vi "Mode to ROI conversion.vi"(10 "Mode":dbl, 11 "Color":string) -> (3 "CCD ROI":cluster{i32, i32, i32, i32, i32, i32}={0, 4096, 1, 0, 4096, 1})   [LabVIEW 2015]
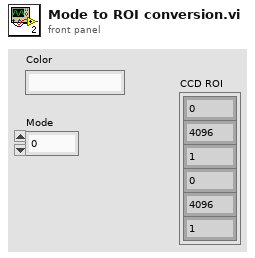
[diagram p1: front panel]
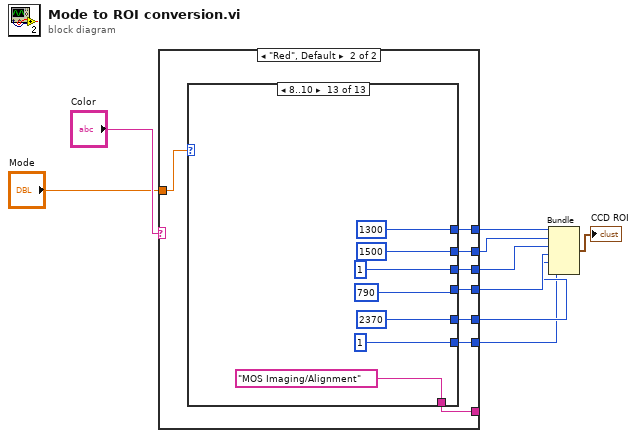
[diagram p0: block diagram]
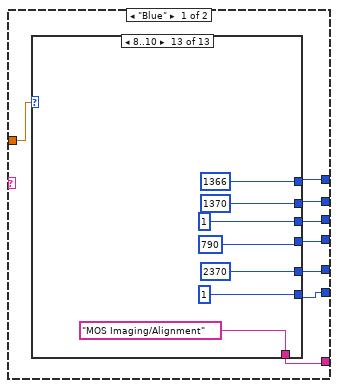
[diagram p2: hidden frame]
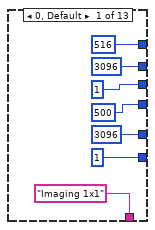
[diagram p3: hidden frame]
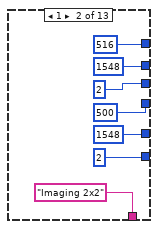
[diagram p4: hidden frame]
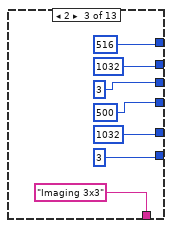
[diagram p5: hidden frame]
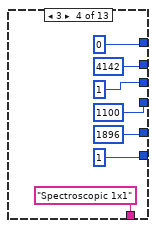
[diagram p6: hidden frame]
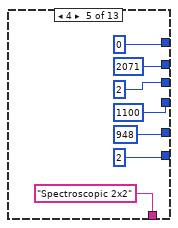
[diagram p7: hidden frame]
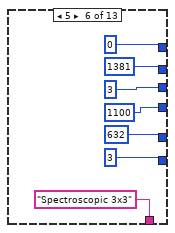
[diagram p8: hidden frame]
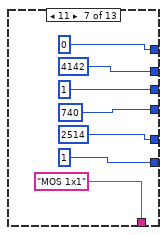
[diagram p9: hidden frame]
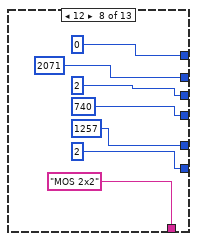
[diagram p10: hidden frame]
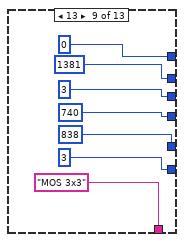
[diagram p11: hidden frame]
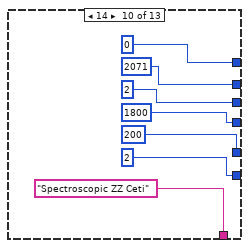
[diagram p12: hidden frame]
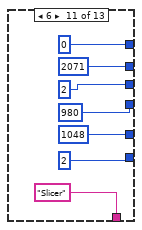
[diagram p13: hidden frame]
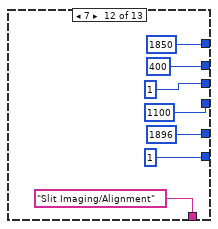
[diagram p14: hidden frame]
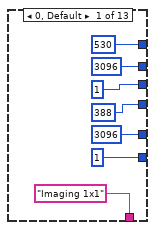
[diagram p15: hidden frame]
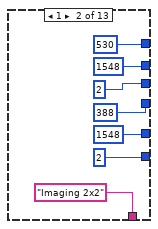
[diagram p16: hidden frame]
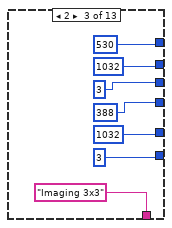
[diagram p17: hidden frame]
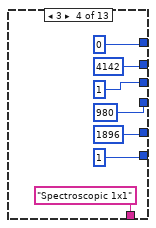
[diagram p18: hidden frame]
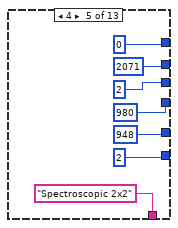
[diagram p19: hidden frame]
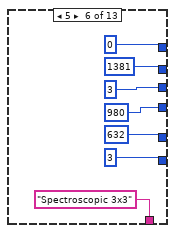
[diagram p20: hidden frame]
diagram:
  n1 = case shown="\"Red\", Default" "Color" {
    tunnel: [w14 w116] -> w6
    tunnel: [w13 w115] -> w5
    tunnel: [w12 w114] -> w4
    tunnel: [w11 w113] -> w3
    tunnel: [w15 w112] -> w2
    tunnel: [w16 w111] -> w1
    tunnel: [w17 w110] -> _
    tunnel: "Mode" -> [w10 w109]
    frame "Blue" {
      n2 = case shown="8..10" w10 {
        tunnel: [516 516 516 0 0 0 0 0 0 0 0 1850 1366] -> w14
        tunnel: [3096 1548 1032 4142 2071 1381 4142 2071 1381 2071 2071 400 1370] -> w13
        tunnel: [1 2 3 1 2 3 1 2 3 2 2 1 1] -> w12
        tunnel: [500 500 500 1100 1100 1100 740 740 740 1800 980 1100 790] -> w11
        tunnel: [3096 1548 1032 1896 948 632 2514 1257 838 200 1048 1896 2370] -> w15
        tunnel: [1 2 3 1 2 3 1 2 3 2 2 1 1] -> w16
        tunnel: ["Imaging 1x1" ("Current Status") "Imaging 2x2" ("Current Status") "Imaging 3x3" ("Current Status") "Spectroscopic 1x1" ("Current Status") "Spectroscopic 2x2" ("Current Status") "Spectroscopic 3x3" ("Current Status") "MOS 1x1" ("Current Status") "MOS 2x2" ("Current Status") "MOS 3x3" ("Current Status") "Spectroscopic ZZ Ceti" ("Current Status") "Slicer" ("Current Status") "Slit Imaging/Alignment" ("Current Status") "MOS Imaging/Alignment" ("Current Status")] -> w17
        frame 0, Default {
        }
        frame 1 {
        }
        frame 2 {
        }
        frame 3 {
        }
        frame 4 {
        }
        frame 5 {
        }
        frame 11 {
        }
        frame 12 {
        }
        frame 13 {
        }
        frame 14 {
        }
        frame 6 {
        }
        frame 7 {
        }
        frame 8..10 {
        }
      }
    }
    frame "Red", Default {
      n3 = case shown="8..10" w109 {
        tunnel: [530 530 530 0 0 0 0 0 0 0 0 1300 1300] -> w116
        tunnel: [3096 1548 1032 4142 2071 1381 4142 2071 1381 2071 2071 1500 1500] -> w115
        tunnel: [1 2 3 1 2 3 1 2 3 2 2 1 1] -> w114
        tunnel: [388 388 388 980 980 980 650 650 650 1800 900 1100 790] -> w113
        tunnel: [3096 1548 1032 1896 948 632 2514 1257 838 200 1048 1896 2370] -> w112
        tunnel: [1 2 3 1 2 3 1 2 3 2 2 1 1] -> w111
        tunnel: ["Imaging 1x1" ("Current Status") "Imaging 2x2" ("Current Status") "Imaging 3x3" ("Current Status") "Spectroscopic 1x1" ("Current Status") "Spectroscopic 2x2" ("Current Status") "Spectroscopic 3x3" ("Current Status") "MOS 1x1" ("Current Status") "MOS 2x2" ("Current Status") "MOS 3x3" ("Current Status") "Spectroscopic ZZ Ceti" ("Current Status") "Slicer" ("Current Status") "Slit Imaging/Alignment" ("Current Status") "MOS Imaging/Alignment" ("Current Status")] -> w110
        frame 0, Default {
        }
        frame 1 {
        }
        frame 2 {
        }
        frame 3 {
        }
        frame 4 {
        }
        frame 5 {
        }
        frame 11 {
        }
        frame 12 {
        }
        frame 13 {
        }
        frame 14 {
        }
        frame 6 {
        }
        frame 7 {
        }
        frame 8..10 {
        }
      }
    }
  }
  n4 = Bundle(w6, w5, w4, w3, w2, w1) -> (→"CCD ROI":cluster{i32, i32, i32, i32, i32, i32})  [unwired: 1 in]
